vi "Step-3-state-index.vi"(11 "2 x U64":u64[](array[numeric]) format="%.0x") -> (3 "j":u64)   [LabVIEW 2017]
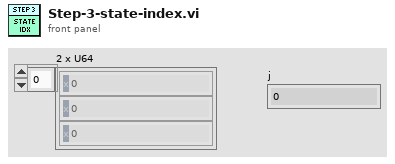
[diagram p1: front panel]
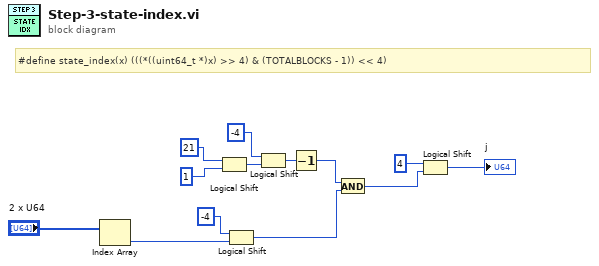
[diagram p0: block diagram]
diagram:
  # "#define state_index(x) (((*((uint64_t *)x) >> 4) & (TOTALBLOCKS - 1)) << 4)"
  n1 = Index Array(array="2 x U64") -> (element=w1:u64)  [unwired: 1 in]
  n2 = Logical Shift(y=i16 21, x=1) -> (x << y=w10:i32)
  n3 = Logical Shift(y=i16 -4, x=w1) -> (x << y=w3:u64)
  n4 = Logical Shift(y=i16 -4, x=w10) -> (x << y=w12:i32)
  n5 = Decrement(x=w12) -> (x-1=w8:i32)
  n6 = And(x=w8, y=w3) -> (x .and. y?=w9:u64)
  n7 = Logical Shift(y=i16 4, x=w9) -> (x << y=→"j":u64)
